vi "Chemical Infuser.vi"(7 "Speed Upgrades":u32 max=8, 9 "Gas B (mB/t)":ext, 10 "Gas A (mB/t)":ext, 11 "Recipe":u16(ring) items=["Sulfur Trioxide", "Sulfuric Acid", "Uranium Hexafluoride"]) -> (0 "Limiting":bool, 1 "B Limiting":bool, 2 "A Limiting":bool, 3 "Output Gas (mB/t)":ext)   [LabVIEW 2023]
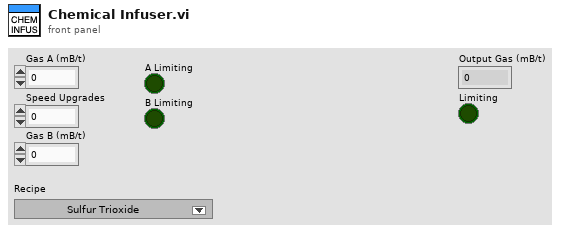
[diagram p1: front panel]
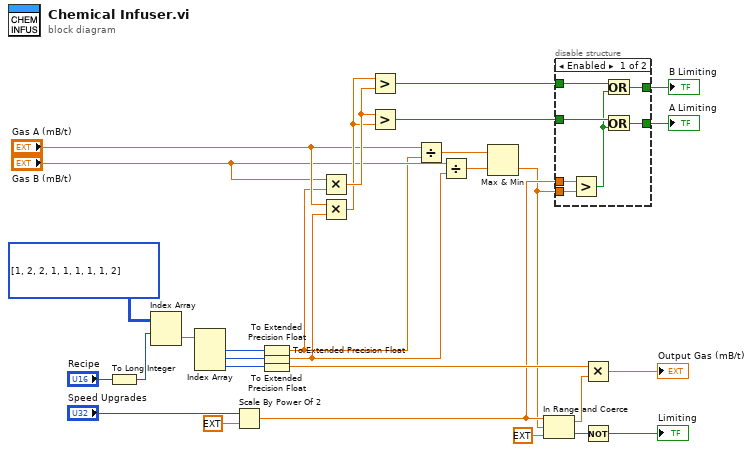
[diagram p0: block diagram]
diagram:
  n1 = To Long Integer(number="Recipe") -> (32bit integer=w20:i32)
  n2 = Index Array(array=u32[][] [[1, 2, 2], [1, 1, 1], [1, 1, 2]], index (row)=w20) -> (element=w18:u32[])  [unwired: 1 in]
  n3 = Index Array(array=w18) -> (element #1=w17:u32, element #2=w3:u32, element #3=w13:u32)  [unwired: 3 in]
  n4 = Scale By Power Of 2(n="Speed Upgrades", x=ext 1.0) -> (x*2^n=w9:ext)
  n5 = To Extended Precision Float(1:w17) -> (0:w4:ext)
  n6 = To Extended Precision Float(1:w3) -> (0:w2:ext)
  n7 = To Extended Precision Float(1:w13) -> (0:w11:ext)
  n8 = Multiply(x="Gas B (mB/t)", y=w4) -> (x*y=w29:ext)
  n9 = Multiply(x="Gas A (mB/t)", y=w2) -> (x*y=w28:ext)
  n10 = Greater?(x=w28, y=w29) -> (0:w23:bool)
  n11 = Greater?(x=w29, y=w28) -> (0:w22:bool)
  n12 = Divide(x="Gas A (mB/t)", y=w4) -> (x/y=w16:ext)
  n13 = Divide(x="Gas B (mB/t)", y=w2) -> (x/y=w15:ext)
  n14 = Max & Min(x=w16, y=w15) -> (min(x,y)=w8:ext)  [unwired: 1 out]
  n15 = In Range and Coerce(upper limit=w9, x=w8, lower limit=ext 0.0) -> (coerced(x)=w12:ext, In Range?=w25:bool)
  n16 = disable-structure shown="Enabled" {
    disable-tunnel: w23 -> [w36 w38]
    disable-tunnel: w22 -> [w35 w37]
    disable-tunnel: [w34 w37] -> w10
    disable-tunnel: w9 -> [w33 _]
    disable-tunnel: w8 -> [w32 _]
    disable-tunnel: [w31 w38] -> w7
    frame Enabled {
      n17 = Greater?(x=w33, y=w32) -> (0:w30:bool)
      n18 = Or(x=w36, y=w30) -> (x .or. y?=w31:bool)
      n19 = Or(x=w35, y=w30) -> (x .or. y?=w34:bool)
    }
    frame Disabled {
    }
  }
  "B Limiting" <- w7
  "A Limiting" <- w10
  n20 = Multiply(x=w11, y=w12) -> (x*y=→"Output Gas (mB/t)":ext)
  n21 = Not(x=w25) -> (.not. x?=→"Limiting":bool)
